vi "Convert to U32.vi"(9 "input valid":bool, 10 "IQData in":T1) -> (1 "output valid":bool, 2 "U32 out":u32, 5 "overflow":bool)   [LabVIEW 2015, in "DDC_7976R_v1.lvlib"]
uses:
  DDC_7976R_v1.lvlib
  <instrlib>/_niInstr/DSP/v1/Shared/Public/IQ Data.ctl
  <vilib>/rvi/FXPMathLib/FxpConvert/subVIs/nifxpmath_Convert_SimConfig.ctl
  <vilib>/fxp/LVFixedPointQuantizationPolicyTypeDef.ctl
  <vilib>/fxp/LVFixedPointOverflowPolicyTypeDef.ctl
  <vilib>/rvi/FXPMathLib/FxpConvert/simVIs/DllFxpConvertTemp_sub.vi
  <vilib>/rvi/FXPMathLib/FxpConvert/XNode/nifxpmath_Convert.xnode
  <instrlib>/_niInstr/DSP/v1/Shared/niInstr DSP v1 Shared.lvlib
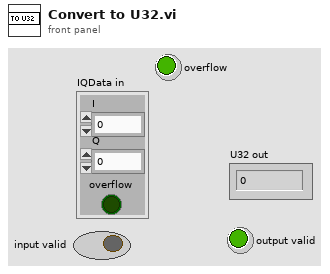
[diagram p1: front panel]
types:
  T1 = typedef "niInstr DSP v1 Shared.lvlib/IQ Data.ctl" = cluster{"I":fxp<+/-,18,1>, "Q":fxp<+/-,18,1>, "overflow":bool}
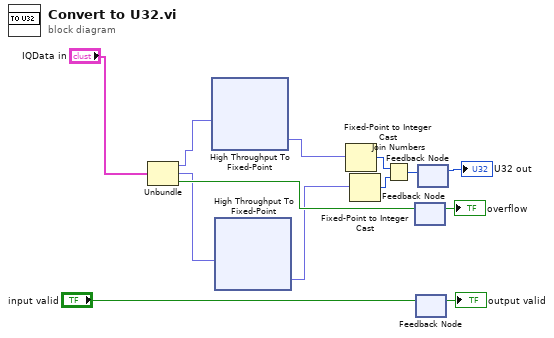
[diagram p0: block diagram]
diagram:
  n1 = Unbundle("IQData in") -> ("I"=w7:fxp<+/-,18,1>, "Q"=w6:fxp<+/-,18,1>, "overflow"=w11:bool)
  n2 = xnode ("High Throughput To Fixed-Point")("x"=w7) -> ("y"=w5:fxp<+/-,16,1>)
  n3 = xnode ("High Throughput To Fixed-Point")("x"=w6) -> ("y"=w4:fxp<+/-,16,1>)
  n4 = Fixed-Point to Integer Cast(1:w5) -> (0:w9:i16)
  n5 = Fixed-Point to Integer Cast(1:w4) -> (0:w8:i16)
  n6 = Join Numbers(hi=w9, lo=w8) -> ((hi.lo)=w13:u32)
  n7 = feedback #1() -> (→"overflow":bool)  [unwired: 1 in]
  n8 = feedback-in #1(w11) -> ()
  n9 = feedback #2() -> (→"output valid":bool)  [unwired: 1 in]
  n10 = feedback-in #2("input valid") -> ()
  n11 = feedback #3() -> (→"U32 out":u32)  [unwired: 1 in]
  n12 = feedback-in #3(w13) -> ()
